vi "GEOM_NOAOCalculateHeadersME.vi"(0 "datacols":i32, 1 "ampxstart":i32, 2 "ampystart":i32, 3 "Corrected ROI":T2={"xstart"=1, "ystart"=1, "xsize"=1, "ysize"=1}, 4 "ampID":string, 5 "datarows":i32, 7 "Requested ROIs":T1(array[cluster]), 9 "overscan":i32, 11 "trims":i32, 12 "bias skip begining":u16, 13 "Binning":cluster{"x":u32, "y":u32}={"x"=1, "y"=1} {"y" min=1; "x" min=1}, 14 "type":u16(ring) items=["LL", "LR", "UL", "UR"], 15 "ytrims":i32) -> (6 "ME Headers out":string[][](table)=[["AMPSEC", "[1:2048,1:4096]", "amplifier section", "STRING"], ["CCDSEC", "[1:2048,1:4096]", "ccd section", "STRING"], ["CCDSIZE", "[1:2048,1:4096]", "ccd size", "STRING"], ["TRIMSEC", "[1:2048,1:4096]", "trim section", "STRING"], ["DATASEC", "[1:2048,1:4096]", "data section", "STRING"], ["BIASSEC", "", "bias section", "STRING"], ["DETSEC", "[14449:16496,24727:28822]", "detector section", "STRING"], ["AMPID", "", "amplifiers ID", "STRING"]], 8 "biassec":string, 10 "detsec":string)   [LabVIEW 2016]
uses:
  GEOM_VAR_action.ctl
panel:
  in  "ME Headers out 2":string[][](table)=[["AMPSEC", "[1:1,1:1]", "amplifier section", "STRING"], ["CCDSEC", "[1:1,1:1]", "ccd section", "STRING"], ["CCDSIZE", "[1:1,1:1]", "ccd size", "STRING"], ["TRIMSEC", "[1:1,1:1]", "trim section", "STRING"], ["DATASEC", "[1:1,1:1]", "data section", "STRING"], ["BIASSEC", "", "bias section", "STRING"], ["DETSEC", "[0:0,0:0]", "detector section", "STRING"], ["AMPID", "", "amplifier id", "STRING"]]
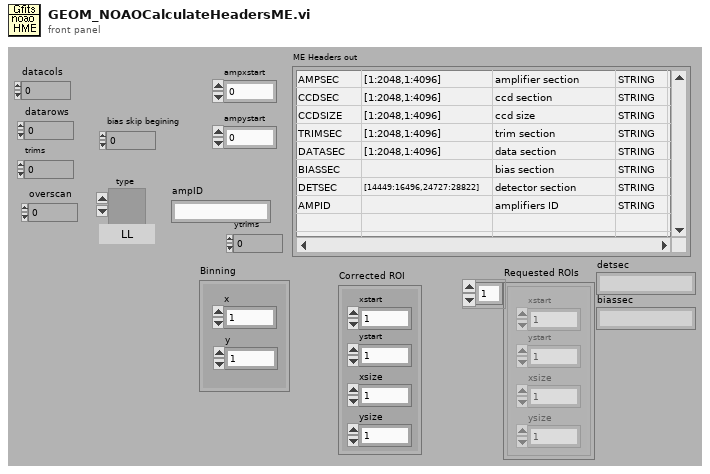
[diagram p1: front panel]
types:
  T1 = cluster{"xstart":u32, "ystart":u32, "xsize":u32, "ysize":u32}[]
  T2 = cluster{"xstart":u32, "ystart":u32, "xsize":u32, "ysize":u32}
  T3 = typedef "GEOM_VAR_action.ctl" = enum16{"read", "write"}
  T4 = typedef "GEOM_CoordsRef.ctl" = cluster{"xref":u32, "yref":u32}
  T5 = cluster{"xstart":i32, "ystart":i32, "xend":i32, "yend":i32}
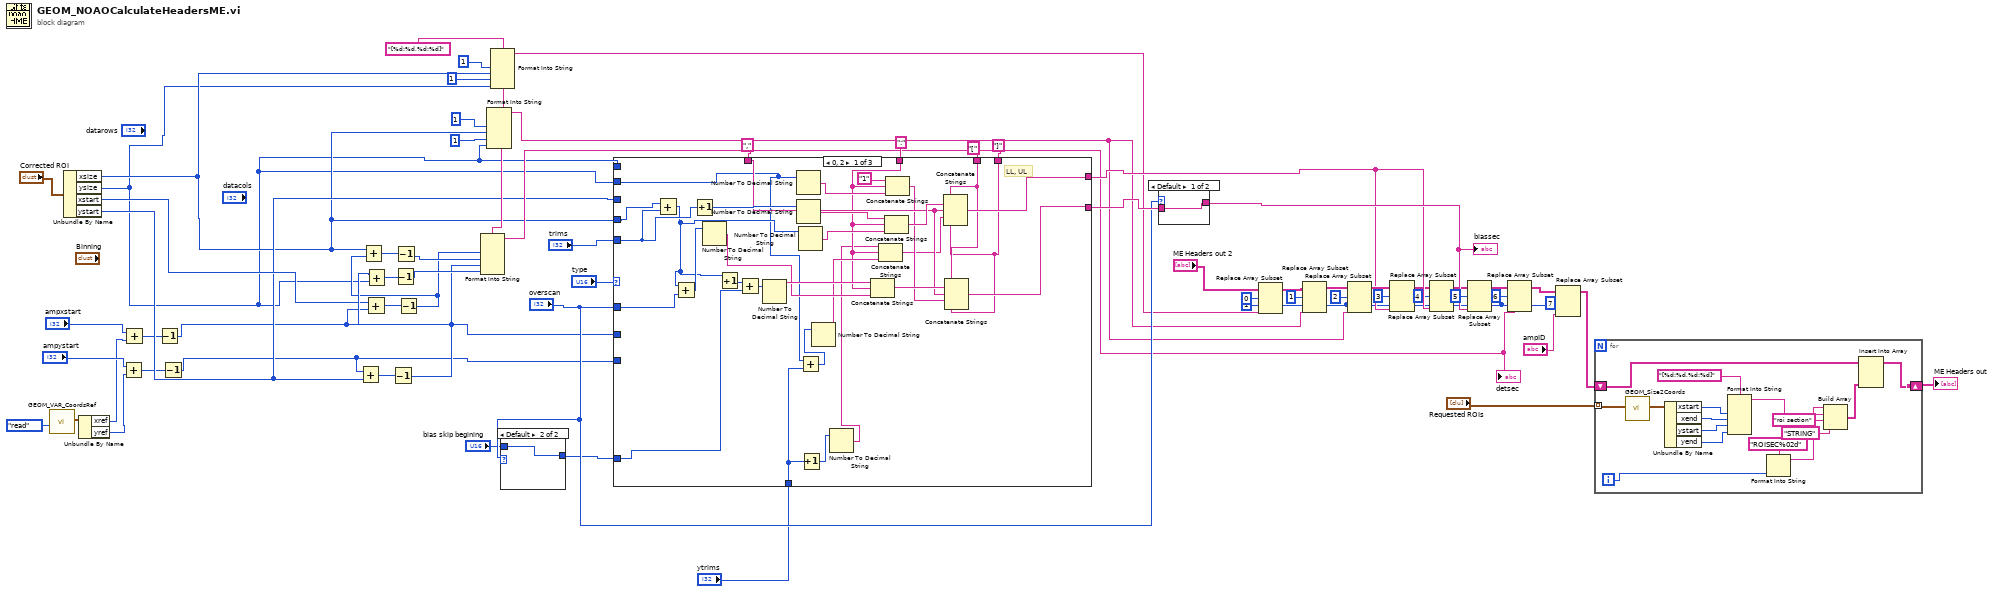
[diagram p0: block diagram]
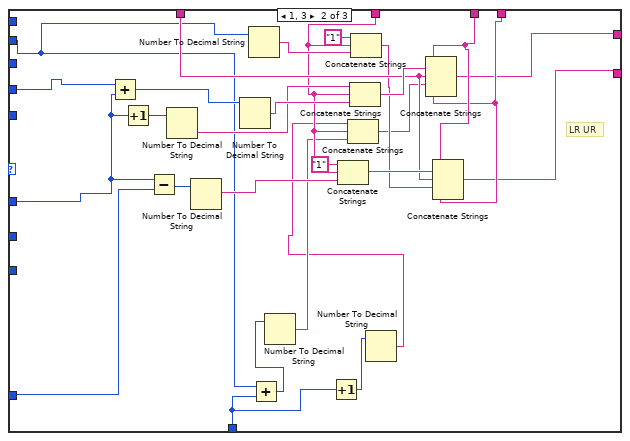
[diagram p2: hidden frame]
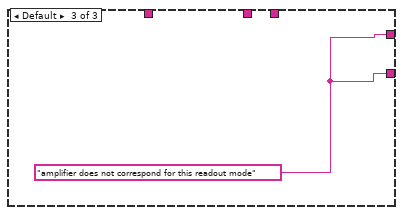
[diagram p3: hidden frame]
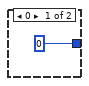
[diagram p4: hidden frame]
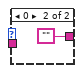
[diagram p5: hidden frame]
diagram:
  w3 = 1 ("disabled index (col)")
  w30 = "[%d:%d,%d:%d]" ("format string")
  n1 = call "GEOM_VAR_CoordsRef.vi"("Action"=GEOM_VAR_action."read") -> ("GEOM_coordsref out"=w10:T4)  [unwired: 1 in, 9 out]
  n2 = Unbundle By Name("Corrected ROI") -> ("xsize"=w21:u32, "ysize"=w20:u32, "xstart"=w23:u32, "ystart"=w22:u32)
  n3 = Unbundle By Name(w10) -> ("xref"=w9:u32, "yref"=w8:u32)
  n4 = Add(x="ampystart", y=w8) -> (x+y=w11:u32)
  n5 = Add(x="ampxstart", y=w9) -> (x+y=w13:u32)
  n6 = Decrement(x=w13) -> (x-1=w7:u32)
  n7 = Decrement(x=w11) -> (x-1=w6:u32)
  n8 = Add(x=w6, y=w22) -> (x+y=w31:u32)
  n9 = Add(x=w23, y=w7) -> (x+y=w32:u32)
  n10 = Decrement(x=w31) -> (x-1=w25:u32)
  n11 = Add(x=w25, y=w20) -> (x+y=w57:u32)
  n12 = Decrement(x=w57) -> (x-1=w58:u32)
  n13 = Decrement(x=w32) -> (x-1=w24:u32)
  n14 = Add(x=w21, y=w24) -> (x+y=w56:u32)
  n15 = Decrement(x=w56) -> (x-1=w55:u32)
  n16 = Format Into String(format string=w30, w24, w55, w25, w58) -> (resulting string=w34:string)  [unwired: 2 in, 1 out]
  "detsec" <- w34
  n17 = Format Into String(format string=w30, 1 ("input 1"), w21, 1 ("input 3"), w20) -> (resulting string=w26:string)  [unwired: 2 in, 1 out]
  n18 = Format Into String(format string=w30, 1 ("input 1"), w21, 1 ("input 3"), w20) -> (resulting string=w27:string)  [unwired: 2 in, 1 out]
  n19 = case shown="Default" "overscan" {
    tunnel: [0 w67] -> w60
    tunnel: "bias skip begining" -> [_ w67]
    frame 0 {
    }
    frame Default {
    }
  }
  n20 = case shown="0, 2" "type" {
    tunnel: [w87 w111 w127] -> w42
    tunnel: w20 -> [_ _ _]
    tunnel: w22 -> [_ _ _]
    tunnel: "trims" -> [w77 _ _]
    tunnel: "overscan" -> [w80 w109 _]
    tunnel: [w92 w110 w127] -> w64
    tunnel: w60 -> [w84 w115 _]
    tunnel: "," ("dim separator") -> [w83 w114 _]
    tunnel: ":" ("pixel separator") -> [w74 w108 _]
    tunnel: "[" -> [w82 w113 _]
    tunnel: "]" -> [w81 w112 _]
    tunnel: w7 -> [_ _ _]
    tunnel: w6 -> [_ _ _]
    tunnel: w20 -> [w69 w103 _]
    tunnel: w21 -> [w78 w104 _]
    tunnel: "ytrims" -> [w70 w101 _]
    frame 0, 2 {
      # "LL, UL"
      n21 = Add(x=w78, y=w77) -> (x+y=w76:u32)
      n22 = Add(x=w76, y=w80) -> (x+y=w93:u32)
      n23 = Increment(x=w77) -> (x+1=w90:i32)
      n24 = Number To Decimal String(number=w93) -> (decimal integer string=w89:string)  [unwired: 1 out]
      n25 = Increment(x=w76) -> (x+1=w85:u32)
      n26 = Add(x=w85, y=w84) -> (x+y=w86:u32)
      n27 = Number To Decimal String(number=w86) -> (decimal integer string=w95:string)  [unwired: 1 out]
      n28 = Number To Decimal String(number=w69) -> (decimal integer string=w97:string)  [unwired: 1 out]
      n29 = Number To Decimal String(number=w90) -> (decimal integer string=w91:string)  [unwired: 1 out]
      n30 = Number To Decimal String(number=w76) -> (decimal integer string=w88:string)  [unwired: 1 out]
      n31 = Add(x=w69, y=w70) -> (x+y=w68:u32)
      n32 = Increment(x=w70) -> (x+1=w72:i32)
      n33 = Number To Decimal String(number=w68) -> (decimal integer string=w75:string)  [unwired: 1 out]
      n34 = Number To Decimal String(number=w72) -> (decimal integer string=w71:string)  [unwired: 1 out]
      n35 = Concatenate Strings(w95, w74, w89) -> (w94:string)
      n36 = Concatenate Strings(w71, w74, w75) -> (w73:string)
      n37 = Concatenate Strings(w91, w74, w88) -> (w96:string)
      n38 = Concatenate Strings("1", w74, w97) -> (w79:string)
      n39 = Concatenate Strings(w82, w96, w83, w73, w81) -> (w87:string)
      n40 = Concatenate Strings(w82, w94, w83, w79, w81) -> (w92:string)
    }
    frame 1, 3 {
      # "LR UR"
      n41 = Add(x=w104, y=w109) -> (x+y=w116:u32)
      n42 = Increment(x=w109) -> (x+1=w118:i32)
      n43 = Subtract(x=w109, y=w115) -> (x-y=w121:i32)
      n44 = Number To Decimal String(number=w118) -> (decimal integer string=w117:string)  [unwired: 1 out]
      n45 = Number To Decimal String(number=w121) -> (decimal integer string=w119:string)  [unwired: 1 out]
      n46 = Number To Decimal String(number=w116) -> (decimal integer string=w124:string)  [unwired: 1 out]
      n47 = Number To Decimal String(number=w103) -> (decimal integer string=w122:string)  [unwired: 1 out]
      n48 = Add(x=w103, y=w101) -> (x+y=w102:u32)
      n49 = Number To Decimal String(number=w102) -> (decimal integer string=w107:string)  [unwired: 1 out]
      n50 = Increment(x=w101) -> (x+1=w100:i32)
      n51 = Concatenate Strings("1" ("Substring"), w108, w119) -> (w125:string)
      n52 = Concatenate Strings(w117, w108, w124) -> (w126:string)
      n53 = Concatenate Strings("1" ("Substring"), w108, w122) -> (w106:string)
      n54 = Number To Decimal String(number=w100) -> (decimal integer string=w99:string)  [unwired: 1 out]
      n55 = Concatenate Strings(w99, w108, w107) -> (w105:string)
      n56 = Concatenate Strings(w113, w126, w114, w105, w112) -> (w111:string)
      n57 = Concatenate Strings(w113, w125, w114, w106, w112) -> (w110:string)
    }
    frame Default {
      w127 = "amplifier does not correspond for this readout mode"
    }
  }
  n58 = case shown="Default" "overscan" {
    tunnel: w64 -> [w128 _]
    tunnel: [w128 ""] -> w63
    frame Default {
    }
    frame 0 {
    }
  }
  "biassec" <- w63
  n59 = Replace Array Subset(array="ME Headers out 2", new element=w27, index (row)=0, index (col)=w3) -> (w35:string[][])
  n60 = Replace Array Subset(array=w35, new element=w26, index (row)=1 ("disabled index (row)"), index (col)=w3) -> (w44:string[][])
  n61 = Replace Array Subset(array=w44, new element=w26, index (row)=2 ("disabled index (row)"), index (col)=w3) -> (w43:string[][])
  n62 = Replace Array Subset(array=w43, new element=w42, index (row)=3 ("disabled index (row)"), index (col)=w3) -> (w41:string[][])
  n63 = Replace Array Subset(array=w41, new element=w42, index (row)=4 ("disabled index (row)"), index (col)=w3) -> (w39:string[][])
  n64 = Replace Array Subset(array=w39, new element=w63, index (row)=5 ("disabled index (row)"), index (col)=w3) -> (w37:string[][])
  n65 = Replace Array Subset(array=w37, new element=w34, index (row)=6 ("disabled index (row)"), index (col)=w3) -> (w5:string[][])
  n66 = Replace Array Subset(array=w5, new element="ampID", index (row)=7, index (col)=w3) -> (w2:string[][])
  n67 = for {
    tunnel: "Requested ROIs" -> [w139] mode=indexing
    shift-right: [w135] -> w18
    shift-left: w2 -> [w138]
    i -> [w136]
    n68 = call "GEOM_Size2Coords.vi"("Size"=w139) -> ("Coords"=w144:T5)  [unwired: 10 out]
    n69 = Unbundle By Name(w144) -> ("xstart"=w143:i32, "xend"=w142:i32, "ystart"=w141:i32, "yend"=w140:i32)
    n70 = Format Into String(format string="[%d:%d,%d:%d]", w143, w142, w141, w140) -> (resulting string=w133:string)  [unwired: 2 in, 1 out]
    n71 = Format Into String(format string="ROISEC%02d", w136) -> (resulting string=w134:string)  [unwired: 2 in, 1 out]
    n72 = Build Array(w134, w133, "roi section" ("element"), "STRING" ("element")) -> (w131:string[])
    n73 = Insert Into Array(array=w138, new element=w131) -> (w135:string[][])  [unwired: 2 in]
  }
  "ME Headers out" <- w18
